vi "Seven Segment Write String.vi"(0 "Arduino Resource":T1={"VISA resource"="", "Board Type"=enum."Uno", "Connection Type"=enum."USB / Serial", "Bytes Per Packet (15)"=15}, 5 "String":string, 9 "Time ms (500)":u32=500, 11 "error in":errorcluster) -> (4 "Arduino Resource":T1={"VISA resource"="", "Board Type"=enum."Uno", "Connection Type"=enum."USB / Serial", "Bytes Per Packet (15)"=15}, 15 "error out":errorcluster)   [LabVIEW 2011, in "LabVIEW Interface for Arduino.lvlib"]
doc: "Write a string to the seven segment display. Arduino Seven Segment Config must be used to configure the seven segment display pins before calling this VI."
uses:
  <vilib>/LabVIEW Interface for Arduino/LabVIEW Interface for Arduino.lvlib
  <vilib>/LabVIEW Interface for Arduino/Private/Type Defs/Arduino Resource.ctl
  <vilib>/LabVIEW Interface for Arduino/Private/Type Defs/Board Type.ctl
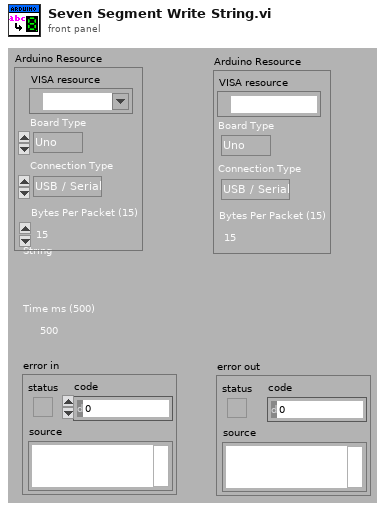
[diagram p1: front panel]
types:
  T1 = typedef "LabVIEW Interface for Arduino.lvlib/Arduino Resource.ctl" = cluster{"VISA resource":refnum<visa-resource-name>, "Board Type":T2, "Connection Type":enum8{"USB / Serial"}, "Bytes Per Packet (15)":u8}
  T2 = typedef "LabVIEW Interface for Arduino.lvlib/Board Type.ctl" = enum16{"Uno", "Dimuelanove w/Atmega 328", "Mega 2560"}
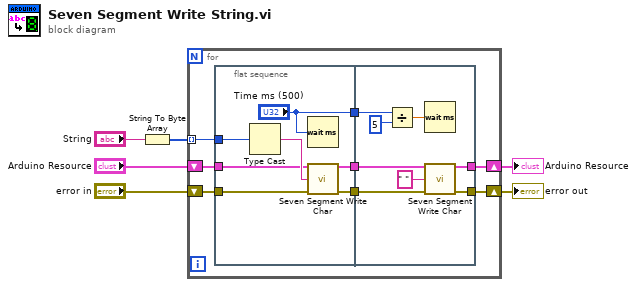
[diagram p0: block diagram]
diagram:
  n1 = String To Byte Array(string="String") -> (unsigned byte array=w5:u8[])
  n2 = for {
    shift-right: [w7] -> w1
    shift-left: "Arduino Resource" -> [w14]
    shift-right: [w12] -> w6
    shift-left: "error in" -> [w13]
    tunnel: w5 -> [w11] mode=indexing
    n3 = flat-sequence {
      tunnel: w14 -> [w16]
      tunnel: w13 -> [w21]
      tunnel: w11 -> [w15]
      tunnel: [w20] -> w10
      tunnel: [w19] -> w9
      tunnel: ["Time ms (500)"] -> w8
      tunnel: [w28] -> w7
      tunnel: [w29] -> w12
      tunnel: w10 -> [w27]
      tunnel: w9 -> [w22]
      tunnel: w8 -> [w25]
      frame #0 {
        n4 = Type Cast(x=w15) -> (*(type *) &x=w18:string)  [unwired: 1 in]
        n5 = Wait (ms)(milliseconds to wait="Time ms (500)") -> ()  [unwired: 1 out]
        n6 = call <vilib>:"Seven Segment Write Char.vi"("Arduino Resource"=w16, "Character"=w18, "error in (no error)"=w21) -> ("Arduino Resource"=w19:T1, "error out"=w20:errorcluster)  [unwired: 11 in]
      }
      frame #1 {
        n7 = Divide(x=w25, y=u32 5 ("milliseconds to wait")) -> (x/y=w23:dbl)
        n8 = Wait (ms)(milliseconds to wait=w23) -> ()  [unwired: 1 out]
        n9 = call <vilib>:"Seven Segment Write Char.vi"("Arduino Resource"=w22, "Character"=" ", "error in (no error)"=w27) -> ("Arduino Resource"=w28:T1, "error out"=w29:errorcluster)  [unwired: 11 in]
      }
    }
  }
  "error out" <- w6
  "Arduino Resource" <- w1
